vi "Start Recipe.vi"(8 "error in (no error)":errorcluster, 10 "Recipe File":path, 11 "Recipe in":refnum<class "Recipe.lvclass">) -> (0 "error out":errorcluster, 3 "Recipe out":refnum<class "Recipe.lvclass">)   [LabVIEW 2022 SP3, in "Recipe.lvclass"]
uses:
  Recipe.lvclass
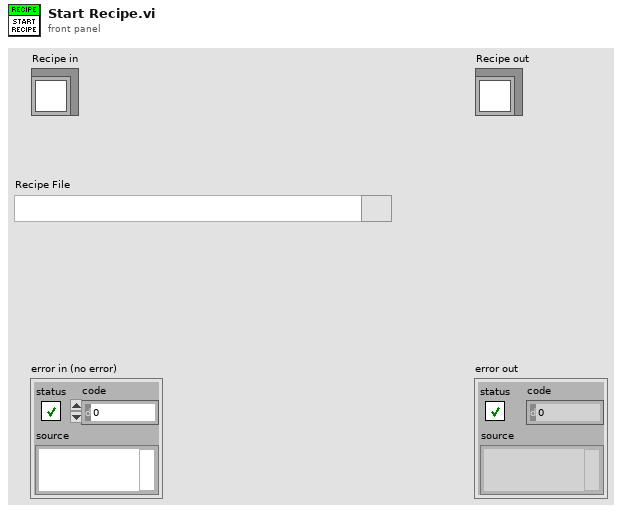
[diagram p1: front panel]
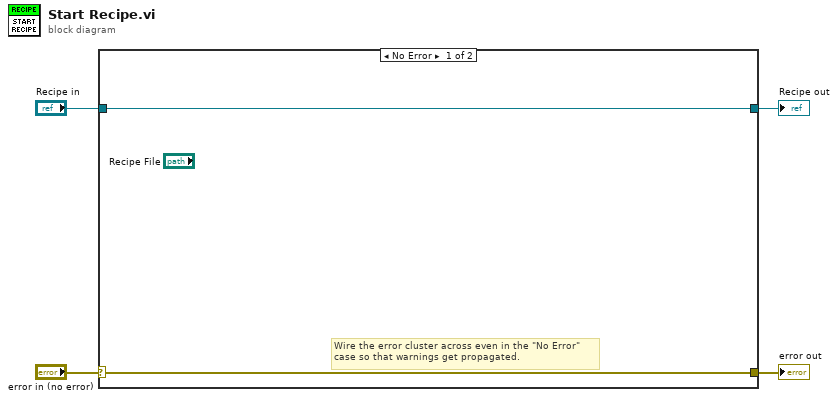
[diagram p0: block diagram]
diagram:
  n1 = case shown="No Error" "error in (no error)" {
    selector: "error in (no error)" -> [w5 w8]
    tunnel: [w5 w8] -> w3
    tunnel: [w6 w7] -> w1
    tunnel: "Recipe in" -> [w6 w7]
    frame No Error {
      # "Wire the error cluster across even in the \"No Error\"\ncase so that warnings get propagated."
    }
    frame Error {
    }
  }
  "error out" <- w3
  "Recipe out" <- w1
